vi "Close.vi"(8 "error in (no error)":errorcluster, 11 "WebSocket in":refnum<class "WebSocket.lvclass">) -> (0 "error out":errorcluster, 3 "WebSocket out":refnum<class "WebSocket.lvclass">)   [LabVIEW 2021, in "WebSockets.lvlib" / "WebSocket.lvclass"]
doc: "Sends the close frame to the WebSocket endpoint and closes the socket connection.\nWebSockets 2.0.1.40\nSam Sharp - MediaMongrels Ltd\nCopyright (c) 2019, MediaMongrels Ltd"
uses:
  WebSocket.lvclass
  WebSocket.lvclass/WebSocket.ctl
  Sockets/Socket/Socket.lvclass
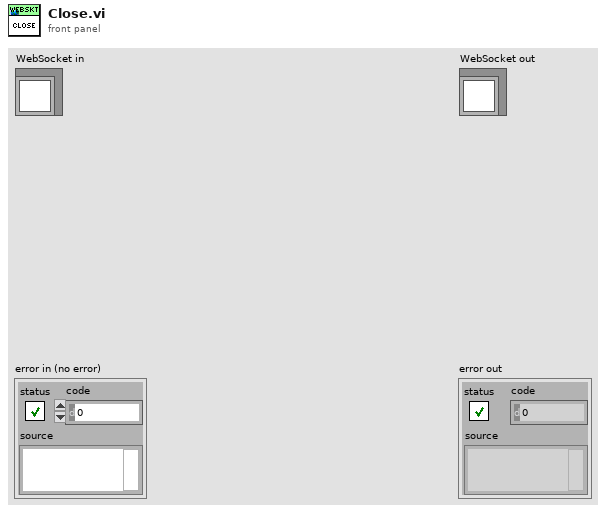
[diagram p1: front panel]
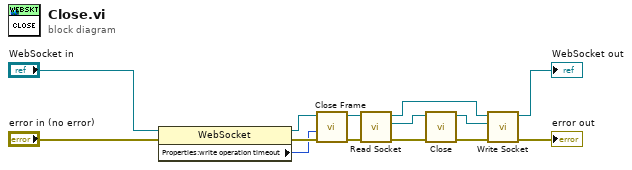
[diagram p0: block diagram]
diagram:
  n1 = property class="WebSocket"(reference="WebSocket in", error in="error in (no error)") -> (reference out=w3:refnum<class "WebSocket.lvclass">, error out=w2:errorcluster, "Properties:write operation timeout"=w1:i32)
  n2 = call-dynamic "Close Frame.vi"("error in (no error)"=w2, "timeout ms (5000)"=w1, "WebSockets in"=w3) -> ("error out"=w13:errorcluster, "WebSockets out"=w14:refnum<class "WebSocket.lvclass">)  [unwired: 7 in]
  n3 = call "Read Socket.vi"("error in (no error)"=w13, "WebSocket in"=w14) -> ("error out"=w11:errorcluster, "Socket"=w12:refnum<class "Socket.lvclass">, "WebSocket out"=w7:refnum<class "WebSocket.lvclass">)  [unwired: 7 in]
  n4 = call-dynamic "Close.vi"("error in (no error)"=w11, "Socket in"=w12) -> ("error out"=w9:errorcluster, "Socket out"=w10:refnum<class "Socket.lvclass">)  [unwired: 8 in]
  n5 = call "Write Socket.vi"("error in (no error)"=w9, "Socket"=w10, "WebSocket in"=w7) -> ("error out"=→"error out":errorcluster, "WebSocket out"=→"WebSocket out":refnum<class "WebSocket.lvclass">)  [unwired: 7 in]
